vi "tester.vi"() -> ()   [LabVIEW 2020]
uses:
  src/path-with-auto-complete.lvclass
panel:
  in  "debug":bool
  in  "Path":path
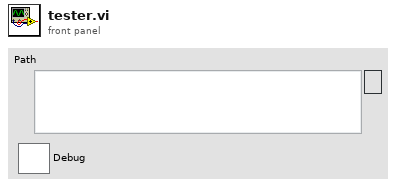
[diagram p1: front panel]
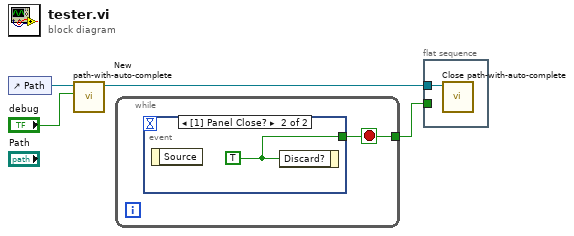
[diagram p0: block diagram]
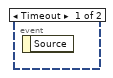
[diagram p2: hidden frame]
diagram:
  n1 = control-ref of="Path"() -> (w4:refnum<vi>)
  n2 = call "New path-with-auto-complete.vi"("debug"="debug", "Reference"=w4) -> ("path-with-auto-complete out"=w2:refnum<class "path-with-auto-complete.lvclass">)  [unwired: 8 in, 1 out]
  n3 = while {
    tunnel: [w5] -> w3
    stop <- w5 stop-if-true
    n4 = event shown="[1] Panel Close?" {
      selector: _ -> [_ _]
      dyn-events: _ -> [_ _]
      timeout: _ -> [_ _]
      tunnel: [_ w6] -> w5
      event Timeout {
        n5 = event-data() -> ()  [unwired: 1 in, 1 out]
      }
      event Panel Close? {
        w6 = TRUE ("Discard?")
        n6 = event-data() -> ()  [unwired: 1 in, 1 out]
        n7 = event-data("Discard?"=w6) -> ()  [unwired: 1 in, 1 out]
      }
    }
  }
  n8 = flat-sequence {
    tunnel: w2 -> [w7]
    tunnel: w3 -> [_]
    frame #0 {
      n9 = call "Close path-with-auto-complete.vi"("path-with-auto-complete in"=w7) -> ()  [unwired: 10 in, 1 out]
    }
  }
